vi "VHM-preLaunchConfig.vi"(10 "preLaunchConfig":T1, 11 "VHM-VNA_Hardware_Manager in":refnum<class "VHM-VNA_Hardware_Manager.lvclass">) -> (3 "VHM-VNA_Hardware_Manager out":refnum<class "VHM-VNA_Hardware_Manager.lvclass">)   [LabVIEW 2020, in "VHM-VNA_Hardware_Manager.lvlib" / "VHM-VNA_Hardware_Manager.lvclass"]
uses:
  VHM-VNA_Hardware_Manager.lvclass
  VHM-preLaunchConfig.ctl
  <vilib>/ActorFramework/Message Enqueuer/Message Enqueuer.lvclass
  VHM-VNA_Hardware_Manager.lvclass/VHM-VNA_Hardware_Manager.ctl
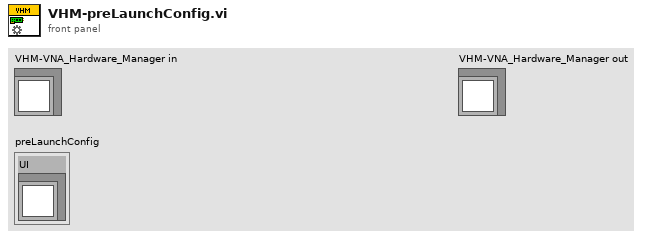
[diagram p1: front panel]
types:
  T1 = typedef "VHM-VNA_Hardware_Manager.lvlib/VHM-VNA_Hardware_Manager.lvclass/VHM-preLaunchConfig.ctl" = cluster{"UI":refnum<class "Message Enqueuer.lvclass">}
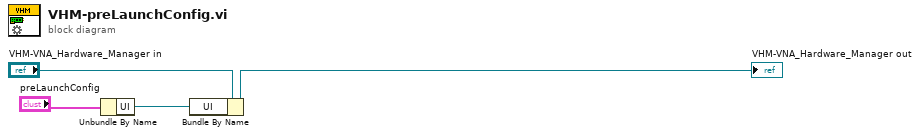
[diagram p0: block diagram]
diagram:
  n1 = Unbundle By Name("preLaunchConfig") -> ("UI"=w1:refnum<class "Message Enqueuer.lvclass">)
  n2 = Bundle By Name(cluster="VHM-VNA_Hardware_Manager in", "UI"=w1) -> (→"VHM-VNA_Hardware_Manager out":refnum<class "VHM-VNA_Hardware_Manager.lvclass">)
